vi "main_transmitter_MIMO_OFDM.vi"() -> ()   [LabVIEW 2020]
uses:
  <instrlib>/niUSRP/niUSRP Timestamp.ctl
  <vilib>/addons/Modulation/Digital/General/MT Generate Bits (Galois, PN Order).vi
  <vilib>/addons/Modulation/Digital/Support/Common/Validators/mod_Generate Bits Validate.vi
  <vilib>/addons/Modulation/Analog/support/mod_Set Error Source.vi
  <instrlib>/niUSRP/niUSRP Configure Time Start Trigger.vi
  <vilib>/addons/Modulation/Digital/General/MT Generate QAM System Parameters(M).vi
  <vilib>/addons/Modulation/Digital/Support/Common/Validators/mod_Generate Filter Coefficients Validate.vi
  <vilib>/addons/Modulation/Digital/General/subVIs/mod_Generate Filter Coefficients.vi
  <vilib>/addons/Modulation/Digital/General/subVIs/mod_Generate Bits PN Sequence.vi
  <vilib>/addons/Modulation/Digital/General/MT Map Bits to QAM Symbols.vi
  <vilib>/addons/Modulation/Digital/General/MT Apply Pulse Shaping Filter (Generic).vi
  <instrlib>/niUSRP/niUSRP Write Tx Data (2D CDB).vi
  <vilib>/addons/Modulation/niDMT.lvlib
panel:
  in  "?":T1(tab)
  in  "start trigger time":T2={"whole seconds"=1, "fractional seconds"=0.1}
  in  "MIMO transmitter (192.168.10.6;192.168.10.7)":refnum<k15>="192.168.10.6;192.168.10.7"
  in  "IQ Rate (915k)":dbl=1000000.0 format="%#_6p"
  in  "Carrier Frequency (2.4G)":dbl=2400000000.0 format="%#_6p"
  in  "TXa Gain (0 to 22)":dbl
  in  "TXa Active Antenna":string="TX1"
  in  "TXb Gain (0 to 22)":dbl
  in  "TXb Active Antenna":string="TX1"
  in  "TXb:Reference Frequency Source (Mimo)":string(combo)="Mimo"
  in  "TXb:Timebase Clock Source (Mimo)":string(combo)="Mimo"
  in  "pulse shaping filter":T3(ring)=enum."Root Raised Cos"
  in  "samples per symbol (16)":i32=4 caption="samples per symbol (4)"
  in  "filter parameter":dbl=0.5 caption="filter parameter (0.5)" format="%.2f"
  in  "filter length (symbols)":i32=8 caption="filter length (8)"
  in  "total bits (128)":i32=512 caption="total bits (512)"
  in  "M-QAM (16)":i32=16
  in  "stop":bool
  out "transmitter error":errorcluster
  out "ERROR":bool
  out "TX error":bool
  out "OFF":bool
  in  "TXa:Reference Frequency Source (Internal)":string(combo)="Internal"
  in  "TXa:Timebase Clock Source (Internal)":string(combo)="Internal"
  in  "FFT Size":u32=256 caption="FFT Size (256)"
  in  "Subcarrier (64)":u32=64
  in  "CP length":u32=32 caption="CP Size (32)"
  out "input bits stream":i8[](array[numeric]) caption="Generated bit stream"
  out "Tramsitted signal (chart)":dbl[][](graph)
  out "Start":bool
  out "Tramsitted signal (graph)":dbl[][](graph)
  out "Packets Sent":i32
  in  "end of data?":bool
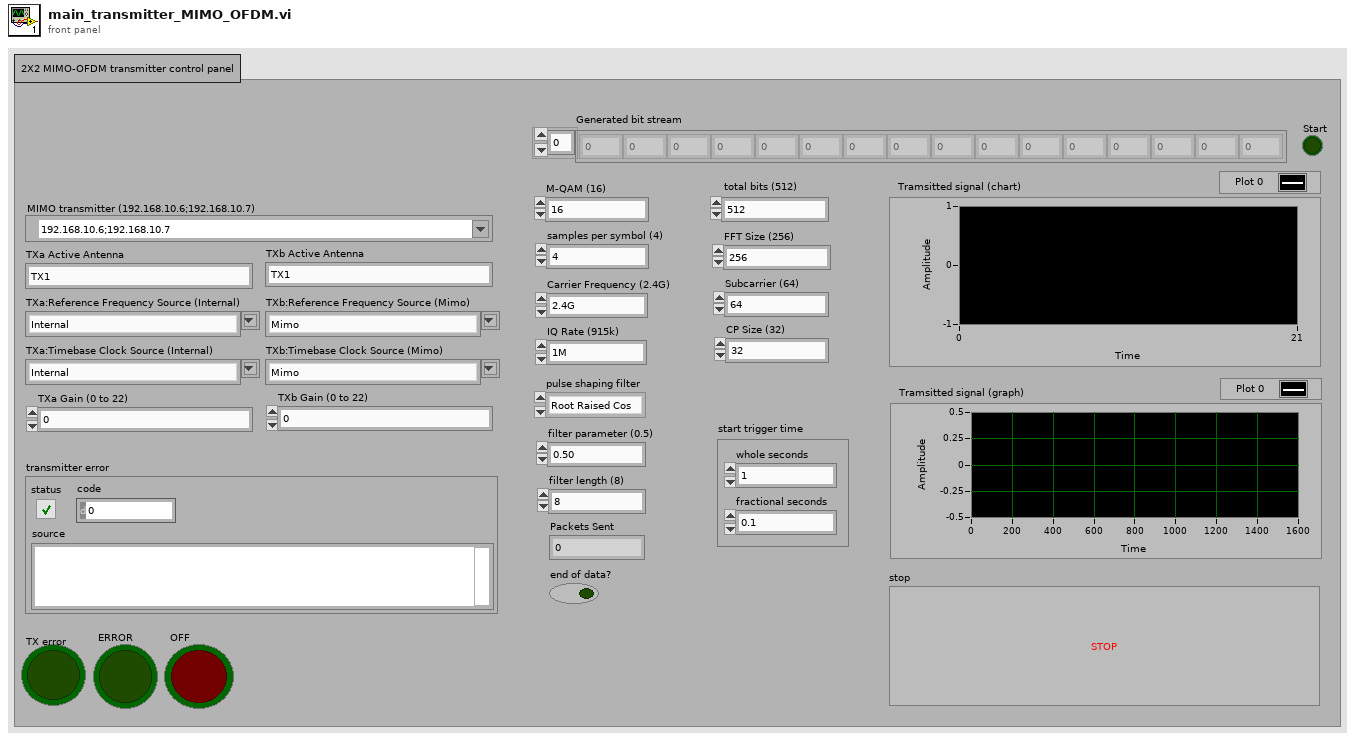
[diagram p1: front panel]
types:
  T1 = enum32{"2X2 MIMO-OFDM transmitter control panel"}
  T2 = typedef "niUSRP Timestamp.ctl" = cluster{"whole seconds":u64, "fractional seconds":dbl}
  T3 = enum16{"none", "Raised Cosine", "Root Raised Cos", "Gaussian"}
  T4 = enum16{"FSK", "PSK", "QAM", "MSK", "PAM", "ASK", "CPM"}
  T5 = cluster{"samples per symbol (16)":i32, "symbol map":cdb[]}
  T6 = typedef "niAMT.lvlib/Complex Data Waveform.ctl" = cluster{"t0":dbl, "dt":dbl, "Y":cdb[]}
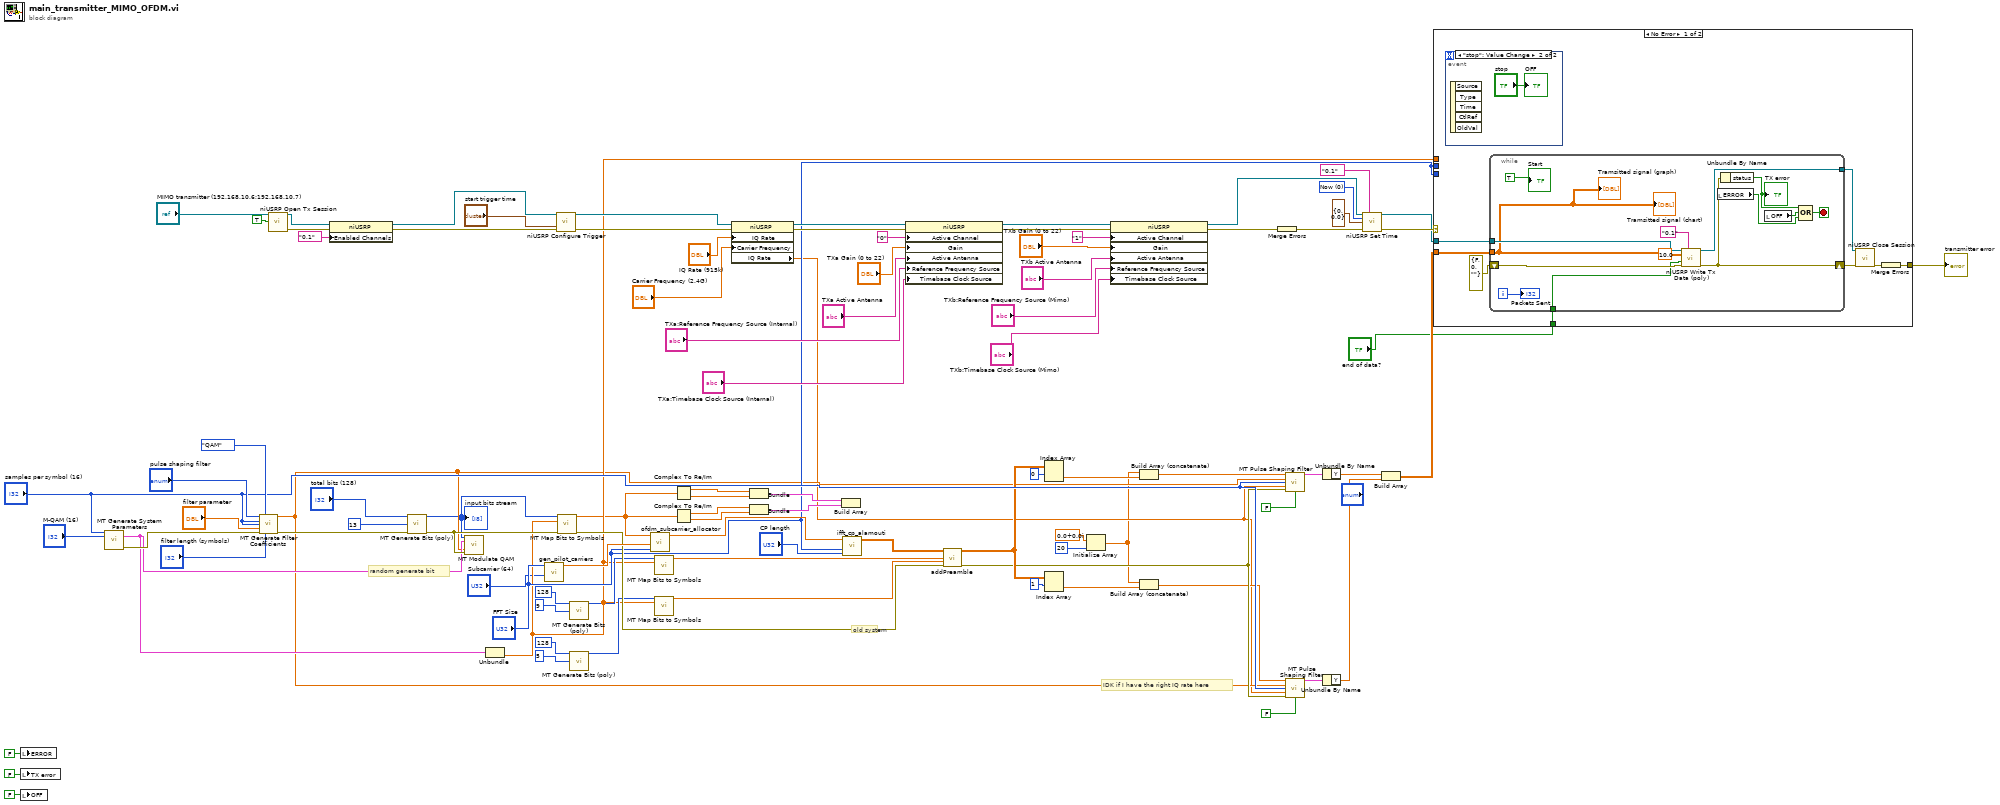
[diagram p0: block diagram]
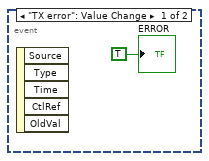
[diagram p2: hidden frame]
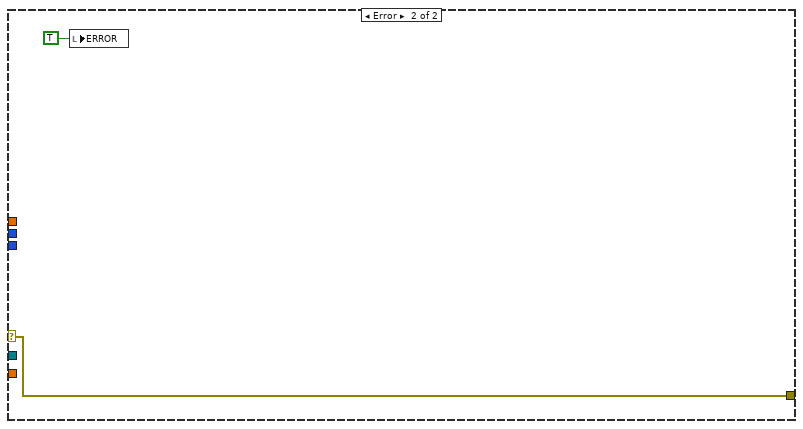
[diagram p3: hidden frame]
diagram:
  w73 = 0 items=["Now", "Next Timebase Edge"] ("apply timestamp")
  # "IDK if I have the right IQ rate here"
  # "old system"
  # "random generate bit"
  n1 = local write "ERROR"(FALSE) -> ()
  n2 = local write "TX error"(FALSE) -> ()
  n3 = local write "OFF"(FALSE) -> ()
  n4 = call-poly <vilib>:"MT Generate System Parameters.vi"("samples per symbol (16)"="samples per symbol (16)", "M-QAM (16)"="M-QAM (16)") -> ("QAM system parameters"=w31:T5, "error out"=w64:errorcluster)  [unwired: 11 in, 1 out]
  n5 = call <vilib>:"MT Generate Filter Coefficients.vi"("pulse shaping filter (none)"="pulse shaping filter", "modulation type"=T4."QAM", "pulse shaping samples per symbol (16)"="samples per symbol (16)", "matched samples per symbol (16)"="samples per symbol (16)", "filter parameter"="filter parameter", "error in (no error)"=w64, "filter length (symbols)"="filter length (symbols)") -> ("pulse shaping filter coefficients"=w23:dbl[], "error out"=w63:errorcluster)  [unwired: 6 in, 1 out]
  n6 = call <instrlib>:"niUSRP Open Tx Session.vi"("device names"="MIMO transmitter (192.168.10.6;192.168.10.7)", "reset"=TRUE) -> ("session handle out"=w52:refnum<k15>, "error out"=w51:errorcluster)  [unwired: 12 in]
  n7 = property class="niUSRP"(reference=w52, error in=w51, "Enabled Channels"="0,1" ("Configuration:Enabled Channels")) -> (reference out=w91:refnum<k15>, error out=w90:errorcluster)
  n8 = call-poly <vilib>:"MT Generate Bits (poly).vi"("total bits (128)"="total bits (128)", "PN sequence order (9)"=13, "error in (no error)"=w63) -> ("output bit stream"=w19:i8[], "error out"=w45:errorcluster)  [unwired: 10 in, 1 out]
  "input bits stream" <- w19
  n9 = call <vilib>:"MT Modulate QAM.vi"("input bit stream"=w19, "QAM system parameters"=w31, "pulse shaping filter coefficients"=w23, "error in (no error)"=w45) -> ()  [unwired: 9 in, 3 out]
  n10 = Unbundle(w31) -> ("symbol map"=w26:cdb[])  [unwired: 1 out]
  n11 = call "gen_pilot_carriers.vi"("message carrier"="Subcarrier (64)", "FFT size"="FFT Size") -> ("TX pilot carriers"=w44:cdb[])  [unwired: 8 in, 1 out]
  n12 = call-poly <instrlib>:"niUSRP Configure Trigger.vi"("session handle"=w91, "start trigger time"="start trigger time", "error in (no error)"=w90) -> ("session handle out"=w89:refnum<k15>, "error out"=w88:errorcluster)  [unwired: 11 in]
  n13 = call-poly <vilib>:"MT Map Bits to Symbols.vi"("input bit stream"=w19, "symbol map"=w26, "error in (no error)"=w45) -> ("symbols"=w20:cdb[], "error out"=w34:errorcluster)  [unwired: 11 in]
  n14 = call-poly <vilib>:"MT Generate Bits (poly).vi"("total bits (128)"=128, "PN sequence order (9)"=9) -> ("output bit stream"=w28:i8[])  [unwired: 11 in, 2 out]
  n15 = call-poly <vilib>:"MT Generate Bits (poly).vi"("total bits (128)"=128, "PN sequence order (9)"=5) -> ("output bit stream"=w30:i8[])  [unwired: 11 in, 2 out]
  n16 = call "ofdm_subcarrier_allocator.vi"("fft size"="FFT Size", "pilot symbol"=w44, "message symbol"=w20) -> ("OFDM symbol"=w43:cdb[])  [unwired: 8 in]
  n17 = call-poly <vilib>:"MT Map Bits to Symbols.vi"("input bit stream"=w28, "symbol map"=w26) -> ("symbols"=w21:cdb[])  [unwired: 12 in, 1 out]
  n18 = call-poly <vilib>:"MT Map Bits to Symbols.vi"("input bit stream"=w30, "symbol map"=w26) -> ("symbols"=w22:cdb[])  [unwired: 12 in, 1 out]
  n19 = Complex To Re/Im(x + iy=w20) -> (x=w59:dbl[], y=w58:dbl[])
  n20 = Complex To Re/Im(x + iy=w20) -> (x=w57:dbl[], y=w56:dbl[])
  n21 = property class="niUSRP"(reference=w89, error in=w88, "IQ Rate"="IQ Rate (915k)", "Carrier Frequency"="Carrier Frequency (2.4G)") -> (reference out=w85:refnum<k15>, error out=w84:errorcluster, "IQ Rate"=w4:dbl)
  n22 = Bundle(w59, w58) -> (w54:cluster{dbl[], dbl[]})  [unwired: 1 in]
  n23 = Bundle(w57, w56) -> (w55:cluster{dbl[], dbl[]})  [unwired: 1 in]
  n24 = Build Array(w54, w55) -> ()  [unwired: 1 out]
  n25 = call "ifft_cp_alamouti.vi"("CP Length"="CP length", "FFT Size"="FFT Size", "Modulated Stream"=w43) -> ("Baseband Streams"=w36:cdb[][])  [unwired: 8 in]
  n26 = property class="niUSRP"(reference=w85, error in=w84, "Active Channel"="0", "Gain"="TXa Gain (0 to 22)", "Active Antenna"="TXa Active Antenna", "Reference Frequency Source"="TXa:Reference Frequency Source (Internal)", "Timebase Clock Source"="TXa:Timebase Clock Source (Internal)") -> (reference out=w80:refnum<k15>, error out=w79:errorcluster)
  n27 = call "addPreamble.vi"("Input Symbol Stream"=w36, "Training Sequence"=w21, "Training Sequence 2"=w22, "error in (no error)"=w34) -> ("Output Transmit \nPackets"=w35:cdb[][], "error out"=w33:errorcluster)  [unwired: 10 in]
  n28 = Index Array(array=w35, index (row)=0) -> (element=w12:cdb[])  [unwired: 1 in]
  n29 = Index Array(array=w35, index (row)=1) -> (element=w13:cdb[])  [unwired: 1 in]
  n30 = Initialize Array(cdb 0.0+0.0i ("element"), 20 ("dimension size")) -> (w3:cdb[])
  n31 = property class="niUSRP"(reference=w80, error in=w79, "Active Channel"="1", "Gain"="TXb Gain (0 to 22)", "Active Antenna"="TXb Active Antenna", "Reference Frequency Source"="TXb:Reference Frequency Source (Mimo)", "Timebase Clock Source"="TXb:Timebase Clock Source (Mimo)") -> (reference out=w11:refnum<k15>, error out=w71:errorcluster)
  n32 = Build Array (concatenate)(w3, w12) -> (w15:cdb[])
  n33 = Build Array (concatenate)(w3, w13) -> (w14:cdb[])
  n34 = Merge Errors(w71) -> (w70:errorcluster)
  n35 = call-poly <vilib>:"MT Pulse Shaping Filter.vi"("symbols"=w15, "pulse shaping filter coefficients"=w23, "samples per symbol (16)"="samples per symbol (16)", "symbol rate (Hz)"=w4, "error in (no error)"=w33, "reset? (T)"=FALSE) -> ("output complex waveform"=w39:T6)  [unwired: 8 in, 1 out]
  n36 = call-poly <vilib>:"MT Pulse Shaping Filter.vi"("symbols"=w14, "pulse shaping filter coefficients"=w23, "samples per symbol (16)"="samples per symbol (16)", "symbol rate (Hz)"=w4, "error in (no error)"=w33, "reset? (T)"=FALSE) -> ("output complex waveform"=w38:T6)  [unwired: 8 in, 1 out]
  n37 = Unbundle By Name(w39) -> ("Y"=w8:cdb[])
  n38 = Unbundle By Name(w38) -> ("Y"=w37:cdb[])
  n39 = call <instrlib>:"niUSRP Set Time.vi"("session handle"=w11, "channel list"="0,1" ("Configuration:Enabled Channels"), "apply timestamp"=w73, "timestamp"=T2 {"whole seconds"=0, "fractional seconds"=0.0}, "error in (no error)"=w70) -> ("session handle out"=w10:refnum<k15>, "error out"=w69:errorcluster)  [unwired: 9 in]
  n40 = Build Array(w8, w37) -> (w7:cdb[][])
  n41 = case shown="No Error" w69 {
    selector: w69 -> [_ w121]
    tunnel: w10 -> [w102 _]
    tunnel: w7 -> [w103 _]
    tunnel: [w98 w121] -> w2
    tunnel: "FFT Size" -> [_ _]
    tunnel: "FFT Size" -> [_ _]
    tunnel: w26 -> [_ _]
    tunnel: "end of data?" -> [w96 _]
    frame No Error {
      n42 = event shown="[1] \"stop\": Value Change" {
        selector: _ -> [_ _]
        dyn-events: _ -> [_ _]
        timeout: _ -> [_ _]
        event "TX error": Value Change {
          n43 = event-data() -> ()  [unwired: 1 in, 5 out]
          "ERROR" <- TRUE
        }
        event "stop": Value Change {
          n44 = event-data() -> ()  [unwired: 1 in, 5 out]
          "OFF" <- "stop"
        }
      }
      n45 = while {
        tunnel: w103 -> [w108]
        tunnel: w102 -> [w119]
        tunnel: [w118] -> w101
        shift-right: [w116] -> w100
        shift-left: errorcluster {"status"=FALSE, "code"=0, "source"=""} ("error out") -> [w117]
        tunnel: w96 -> [w106]
        i -> [w109]
        stop <- w114 stop-if-true
        n46 = call-poly <instrlib>:"niUSRP Write Tx Data (poly).vi"("session handle"=w119, "channel list"="0,1", "data"=w108, "timeout"=10.0, "end of data?"=w106, "error in (no error)"=w117) -> ("session handle out"=w118:refnum<k15>, "error out"=w116:errorcluster)  [unwired: 8 in]
        n47 = local read "ERROR"() -> (w113:bool)
        n48 = Unbundle By Name(w116) -> ("status"=w115:bool)
        "TX error" <- w115
        n49 = local read "OFF"() -> (w112:bool)
        n50 = Compound Arithmetic op=OR(w115, w112, w113) -> (w114:bool)
        "Tramsitted signal (chart)" <- w108
        "Start" <- TRUE
        "Tramsitted signal (graph)" <- w108
        "Packets Sent" <- w109
      }
      n51 = call <instrlib>:"niUSRP Close Session.vi"("session handle"=w101, "error in (no error)"=w100) -> ("error out"=w99:errorcluster)  [unwired: 13 in]
      n52 = Merge Errors(w99) -> (w98:errorcluster)
    }
    frame Error {
      n53 = local write "ERROR"(TRUE) -> ()
    }
  }
  "transmitter error" <- w2
